vi "Remove Panel.vi"(8 "error in (no error)":errorcluster, 10 "Panel in":refnum<class "ArrayPanel.lvclass">, 11 "ArrayManager in":refnum<class "ArrayManager.lvclass">) -> (0 "error out":errorcluster, 2 "Panel":refnum<class "ArrayPanel.lvclass">, 3 "ArrayManager out":refnum<class "ArrayManager.lvclass">)   [LabVIEW 2020, in "OOPanel.lvlib" / "ArrayManager.lvclass"]
uses:
  ArrayManager.lvclass
  ArrayPanel/ArrayPanel.lvclass
  ArrayManager.lvclass/ArrayManager.ctl
  ArrayPanel/ArrayPanel.lvclass/ArrayPanel.ctl
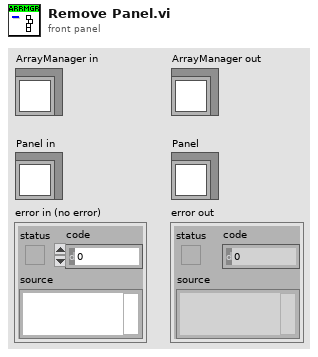
[diagram p1: front panel]
types:
  T1 = typedef "OOPanel.lvlib/ArrayManager.lvclass/State Ref.ctl" = cluster{"Running":bool, "Borders":bool, "Total Height":dbl, "Scroll Visible":bool}
  T2 = typedef "OOPanel.lvlib/ArrayPanel.lvclass/Desired Size.ctl" = cluster{"Width":u32, "Height":u32}
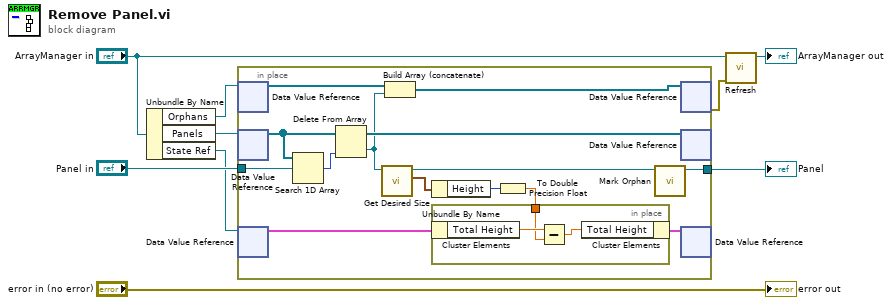
[diagram p0: block diagram]
diagram:
  n1 = Unbundle By Name("ArrayManager in") -> ("Orphans"=w6:refnum<data-value>, "Panels"=w9:refnum<data-value>, "State Ref"=w5:refnum<data-value>)
  n2 = in-place {
    in-place-border: "Panel in" -> [w23]
    in-place-border: [w17] -> w7
    n3 = in-place-dvr #1(w6) -> (w19:refnum<class "ArrayPanel.lvclass">[])  [unwired: 1 out]
    n4 = in-place-dvr #2(w9) -> (w22:refnum<class "ArrayPanel.lvclass">[])  [unwired: 1 out]
    n5 = in-place-dvr #3(w5) -> (w16:T1)  [unwired: 1 out]
    n6 = Search 1D Array(1D array=w22, element=w23) -> (index of element=w21:i32)  [unwired: 1 in]
    n7 = Delete From Array(array=w22, index=w21) -> (deleted portion=w15:refnum<class "ArrayPanel.lvclass">, array with subset deleted=w20:refnum<class "ArrayPanel.lvclass">[])  [unwired: 1 in]
    n8 = call-dynamic "Get Desired Size.vi"("ArrayPanel in"=w15) -> ("Desired Size"=w14:T2, "ArrayPanel out"=w12:refnum<class "ArrayPanel.lvclass">)  [unwired: 8 in, 1 out]
    n9 = Build Array (concatenate)(w19, w15) -> (w18:refnum<class "ArrayPanel.lvclass">[])
    n10 = Unbundle By Name(w14) -> ("Height"=w13:u32)
    n11 = To Double Precision Float(number=w13) -> (double precision float=w11:dbl)
    n12 = in-place {
      in-place-border: w11 -> [w25]
      n13 = in-place-cluster #4(w16) -> ("Total Height"=w26:dbl)
      n14 = Subtract(x=w26, y=w25) -> (x-y=w24:dbl)
      n15 = in-place-cluster #4("Total Height"=w24) -> (w10:T1)
    }
    n16 = call "Mark Orphan.vi"("ArrayPanel in"=w12) -> ("ArrayPanel out"=w17:refnum<class "ArrayPanel.lvclass">)  [unwired: 9 in, 1 out]
    n17 = in-place-dvr #1(w18) -> (w1:errorcluster)  [unwired: 1 out]
    n18 = in-place-dvr #2(w20) -> ()  [unwired: 2 out]
    n19 = in-place-dvr #3(w10) -> ()  [unwired: 2 out]
  }
  "Panel" <- w7
  n20 = call "Refresh.vi"("error in (no error)"=w1, "ArrayManager in"="ArrayManager in") -> ("ArrayManager out"=→"ArrayManager out":refnum<class "ArrayManager.lvclass">)  [unwired: 8 in, 1 out]
  "error out" <- "error in (no error)"
